vi "SetChainLength.vi"(8 "error in (no error)":errorcluster, 10 "Chain Length":u8, 11 "ControlState in":T1 {"ChainMask" format="0x%02x"}) -> (0 "error out":errorcluster, 3 "ControlState out":T1 {"ChainMask" format="0x%02x"})   [LabVIEW 2018, in "ArduinoSerialBling.lvlib"]
uses:
  ArduinoSerialBling.lvlib
  ControlState.ctl
  ConnectionType.ctl
  UdpConnection.ctl
  ChainState.ctl
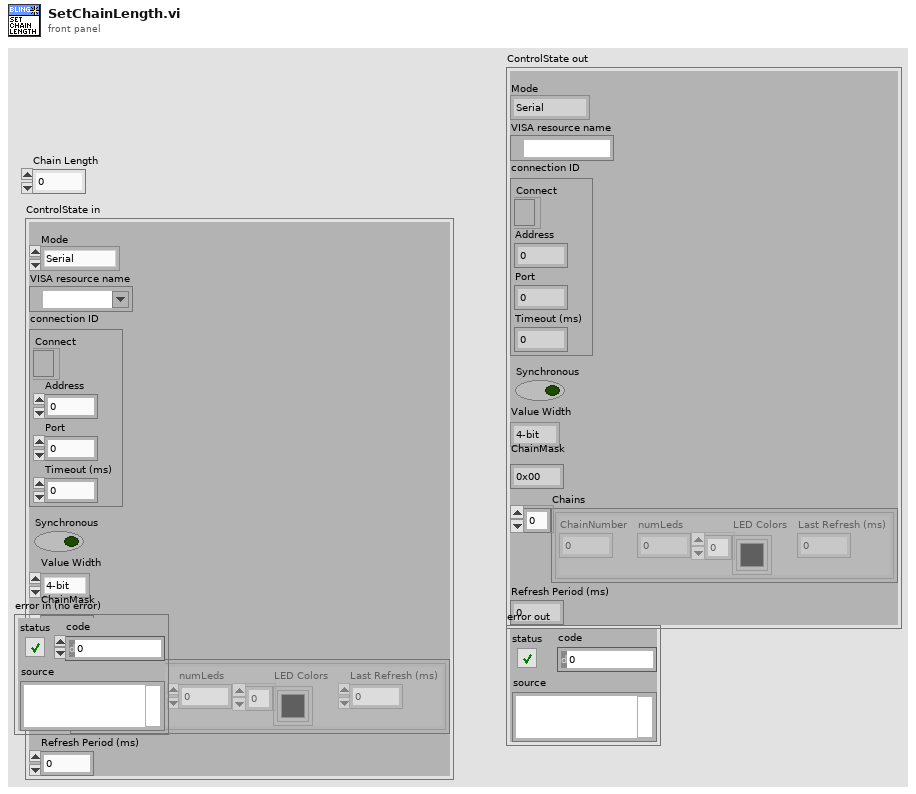
[diagram p1: front panel]
types:
  T1 = typedef "ArduinoSerialBling.lvlib/ControlState.ctl" = cluster{"Mode":T2, "VISA resource name":refnum<visa-resource-name>, "connection ID":T3, "Synchronous":bool, "Value Width":enum16{"4-bit", "8-bit"}, "ChainMask":u8, "Chains":T4[], "Refresh Period (ms)":u32}
  T2 = typedef "ConnectionType.ctl" = enum16{"Serial", "Ethernet", "Offline"}
  T3 = typedef "UdpConnection.ctl" = cluster{"Connect":refnum<k16>, "Address":u32, "Port":u16, "Timeout (ms)":i32}
  T4 = typedef "ArduinoSerialBling.lvlib/ChainState.ctl" = cluster{"ChainNumber":u8, "numLeds":u8, "LED Colors":u32[], "Last Refresh (ms)":u32}
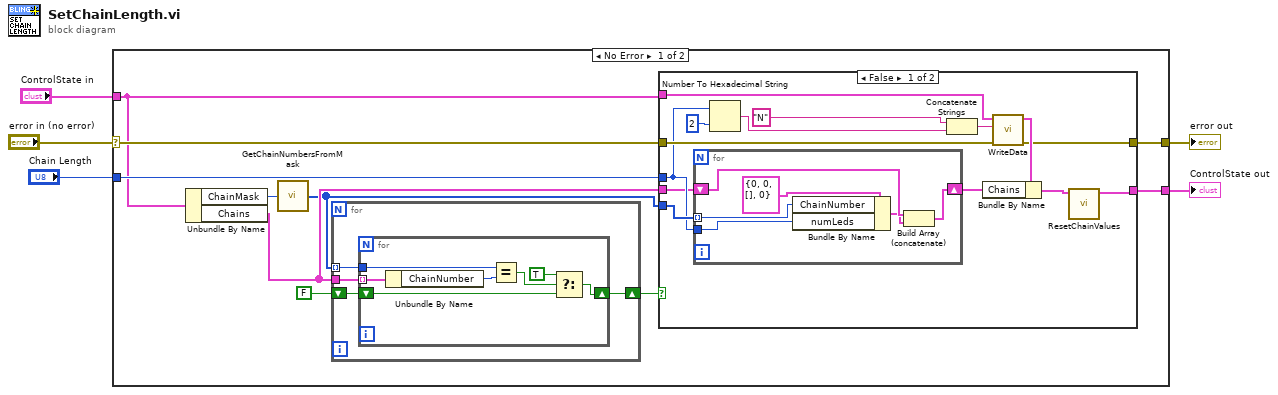
[diagram p0: block diagram]
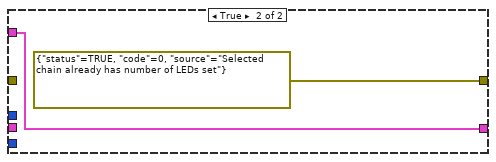
[diagram p2: hidden frame]
diagram:
  n1 = case shown="No Error" "error in (no error)" {
    selector: "error in (no error)" -> [w15 w49]
    tunnel: "ControlState in" -> [w12 w50]
    tunnel: [w11 w50] -> w5
    tunnel: [w14 w49] -> w2
    tunnel: "Chain Length" -> [w13 _]
    frame No Error {
      n2 = Unbundle By Name(w12) -> ("ChainMask"=w7:u8, "Chains"=w9:T4[])
      n3 = call "GetChainNumbersFromMask.vi"("ChainMask"=w7) -> ("Chains"=w6:u8[])
      n4 = for {
        shift-right: [w16] -> w8
        shift-left: FALSE -> [w17]
        tunnel: w9 -> [w19]
        tunnel: w6 -> [w18] mode=indexing
        n5 = for {
          tunnel: w19 -> [w25] mode=indexing
          tunnel: w18 -> [w26]
          shift-right: [w20] -> w16
          shift-left: w17 -> [w22]
          n6 = Unbundle By Name(w25) -> ("ChainNumber"=w24:u8)
          n7 = Equal?(x=w26, y=w24) -> (x = y?=w23:bool)
          n8 = Select(t=TRUE, s=w23, f=w22) -> (s? t:f=w20:bool)
        }
      }
      n9 = case shown="False" w8 {
        tunnel: w15 -> [w34 _]
        tunnel: [w35 errorcluster {"status"=TRUE, "code"=0, "source"="Selected chain already has number of LEDs set"} ("error out")] -> w14
        tunnel: w6 -> [w31 _]
        tunnel: w13 -> [w30 _]
        tunnel: w9 -> [w29 _]
        tunnel: w12 -> [w37 w48]
        tunnel: [w27 w48] -> w11
        frame False {
          n10 = for {
            tunnel: w31 -> [w45] mode=indexing
            tunnel: w30 -> [w44]
            shift-right: [w41] -> w32
            shift-left: w29 -> [w43]
            n11 = Bundle By Name(cluster=T4 {"ChainNumber"=0, "numLeds"=0, "LED Colors"=[], "Last Refresh (ms)"=0} ("ChainState"), "ChainNumber"=w45, "numLeds"=w44) -> (w42:T4)
            n12 = Build Array (concatenate)(w43, w42) -> (w41:T4[])
          }
          n13 = Number To Hexadecimal String(1:i16 2 ("width (-)"), 2:w30) -> (0:w39:string)
          n14 = Concatenate Strings("N", w39) -> (w33:string)
          n15 = call "WriteData.vi"("error in (no error)"=w34, "Command"=w33, "ControlState in"=w37) -> ("error out"=w35:errorcluster, "ControlState out"=w36:T1)  [unwired: 5 in, 2 out]
          n16 = Bundle By Name(cluster=w36, "Chains"=w32) -> (w28:T1)
          n17 = call "ResetChainValues.vi"("ControlState in"=w28) -> ("ControlState out"=w27:T1)  [unwired: 8 in, 2 out]
        }
        frame True {
        }
      }
    }
    frame Error {
    }
  }
  "ControlState out" <- w5
  "error out" <- w2
